vi "Create (Factory).vi"(5 "Sequencing":refnum<class "MessageQ.lvclass">, 6 "Variables":refnum<class "Variables.lvclass">, 7 "VolatusAPI":refnum<class "VolatusAPI.lvclass">, 8 "MultiErrors":refnum<class "MultiErrors.lvclass">, 10 "Transition Config":refnum<class "Transition Config.lvclass">) -> (0 "MultiErrors out":refnum<class "MultiErrors.lvclass">, 3 "Transition out":refnum<class "Transition.lvclass">)   [LabVIEW 2020, in "VolatusSeq.lvlib" / "Transition.lvclass"]
uses:
  Transition.lvclass
  VolatusSeqConfig/Transition Config/Transition Config.lvclass
  Volatus/VolatusAPI/VolatusAPI.lvclass
  VolatusErrorUtilities/MultiErrors/MultiErrors.lvclass
  Volatus/MessageQ/MessageQ.lvclass
  VolatusErrorUtilities/MultiErrors/MultiErrors.lvclass/MultiErrors.ctl
  VolatusErrorUtilities/MultiErrors/Last Error to Wire.vi
  Transition.lvclass/Transition.ctl
  VolatusSeq.lvlib
  Variables/Variables.lvclass
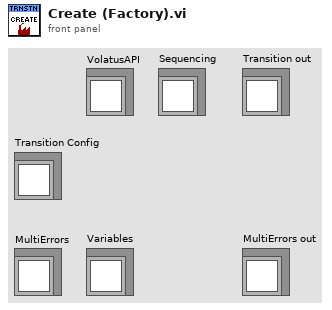
[diagram p1: front panel]
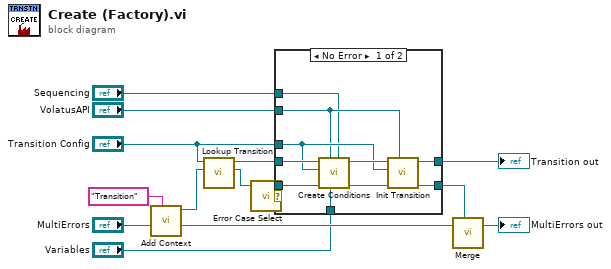
[diagram p0: block diagram]
diagram:
  n1 = call "Add Context.vi"("Context"="Transition", "MultiErrors in"="MultiErrors") -> ("Original Context"=w3:refnum<class "MultiErrors.lvclass">, "Added Context"=w5:refnum<class "MultiErrors.lvclass">)  [unwired: 8 in]
  n2 = call "Lookup Transition.vi"("error in (no error)"=w5, "Transition Config"="Transition Config") -> ("error out"=w8:refnum<class "MultiErrors.lvclass">, "Transition"=w14:refnum<class "Transition.lvclass">)  [unwired: 8 in]
  n3 = call "Error Case Select.vi"("MultiErrors in"=w8) -> ("MultiErrors out"=w6:refnum<class "MultiErrors.lvclass">, "error out"=w7:errorcluster)  [unwired: 7 in]
  n4 = case shown="No Error" w7 {
    tunnel: "VolatusAPI" -> [w20 _]
    tunnel: [w25 _] -> w13
    tunnel: w14 -> [w23 _]
    tunnel: "Transition Config" -> [w21 _]
    tunnel: w6 -> [w19 w26]
    tunnel: [w18 w26] -> w15
    tunnel: "Sequencing" -> [w17 _]
    tunnel: "Variables" -> [w16 _]
    frame No Error {
      n5 = call "Create Conditions.vi"("Sequencing"=w17, "Variables"=w16, "VolatusAPI"=w20, "error in (no error)"=w19, "Transition Config"=w21, "Transition in"=w23) -> ("error out"=w24:refnum<class "MultiErrors.lvclass">, "Transition out"=w22:refnum<class "Transition.lvclass">)  [unwired: 4 in]
      n6 = call-dynamic "Init Transition.vi"("VolatusAPI"=w20, "error in (no error)"=w24, "Transition Config"=w21, "Transition in"=w22) -> ("error out"=w18:refnum<class "MultiErrors.lvclass">, "Transition out"=w25:refnum<class "Transition.lvclass">)  [unwired: 6 in]
    }
    frame Error {
    }
  }
  "Transition out" <- w13
  n7 = call "Merge.vi"("First Error In"=w3, "Second Error In"=w15) -> ("MultiErrors out"=→"MultiErrors out":refnum<class "MultiErrors.lvclass">)  [unwired: 5 in]
